vi "iWorx - Conductivity_.vi"() -> ()   [LabVIEW 2012]
uses:
  <vilib>/DAQmx/read.llb/DAQmx Read (Analog 1D Wfm NChan 1Samp).vi
  <vilib>/DAQmx/create/channels.llb/DAQmx Create Channel (AI-Voltage-Basic).vi
  <vilib>/DAQmx/miscellaneous.llb/DAQmx Fill In Error Info.vi
panel:
  in  "Reset Default Cal":bool
  in  "Set Points":T1={"SP1 Voltage"=0.2, "SP1 Value"=20.0, "SP1 Voltage 2"=2.0, "SP1 Value 2"=200.0} {"SP1 Value 2" format="%.1f mS"; "SP1 Voltage 2" format="%.1f V"; "SP1 Value" format="%.1f mS"; "SP1 Voltage" format="%.1f V"}
  in  "Set Up":bool
  out "Offset":dbl=-1.1111111111111112
  out "Slope":dbl=5.277777777777778
  in  "Channel":u16(ring) items=["Channel 1", "Channel 2"]
  in  "Pause Button":bool
  in  "Snapshot":bool
  out "Processed Signal":dbl(knob) caption="Conductivity" scale=0.0..20.0
  in  "stop":bool
  out "Waveform Chart":waveform(dbl)(graph)
  in  "Sample Timing":u16(ring)=200 items=["20Hz"=50, "5 Hz"=200, "2 Hz"=500, "1 Hz"=1000, ".5 Hz"=2000, ".2 Hz"=5000]
  in  "Clear Chart":bool
  in  "Open Log":bool
  in  "Autoscale Y":bool
  out "Raw Signal":dbl(knob) scale=-10.0..10.0
  # "iWorx - Conductivity Probe - Data Logger"
  # "Sensor Input"
  # "(              ,              )"
  # "(              ,              )"
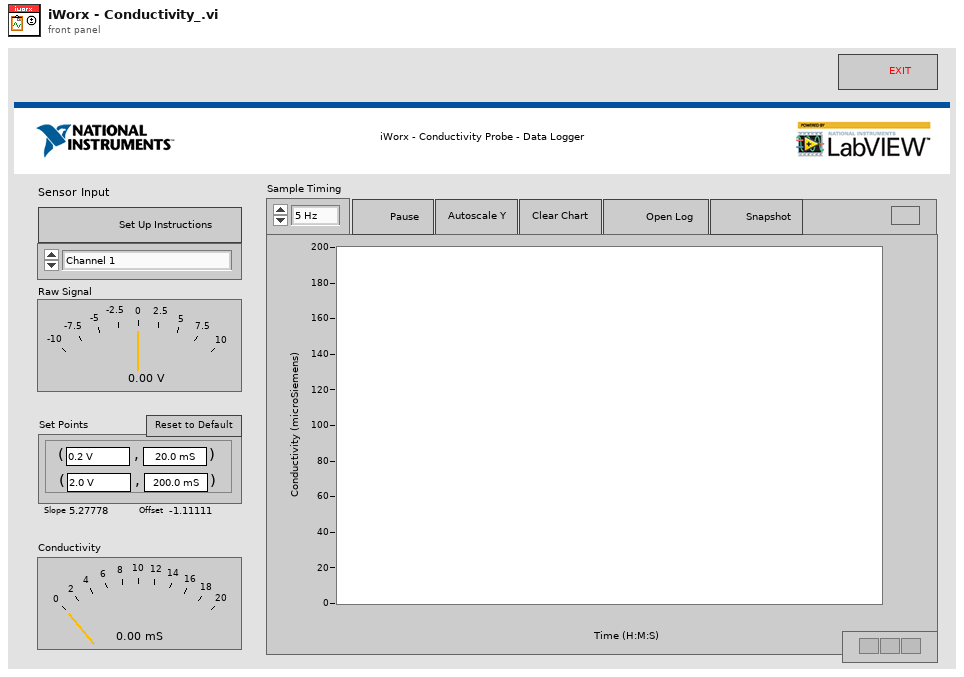
[diagram p1: front panel]
types:
  T1 = cluster{"SP1 Voltage":dbl, "SP1 Value":dbl, "SP1 Voltage 2":dbl, "SP1 Value 2":dbl}
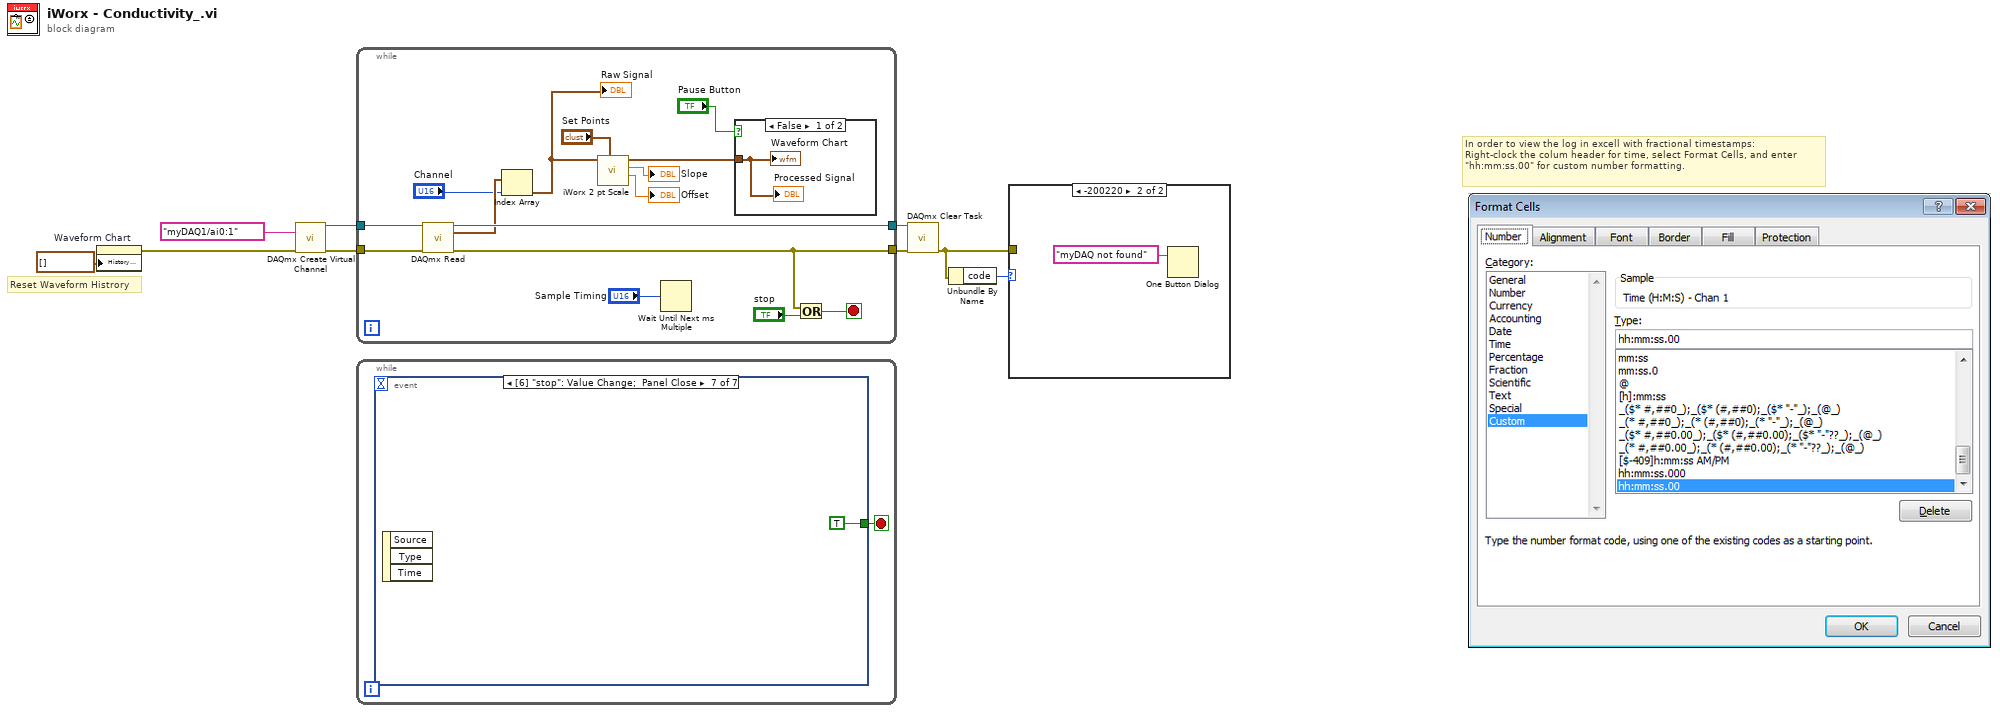
[diagram p0: block diagram]
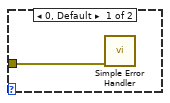
[diagram p2: hidden frame]
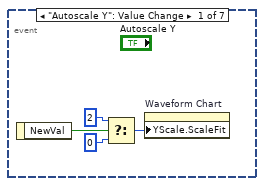
[diagram p3: hidden frame]
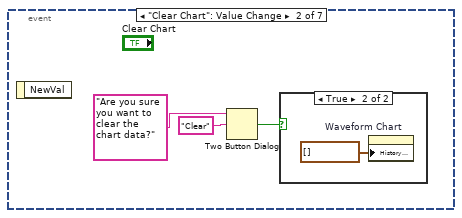
[diagram p4: hidden frame]
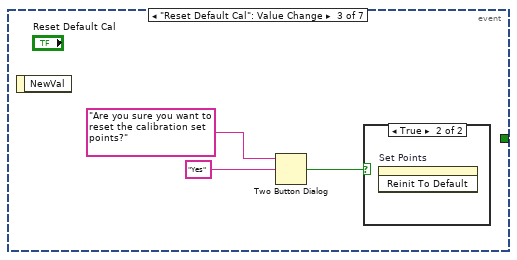
[diagram p6: hidden frame]
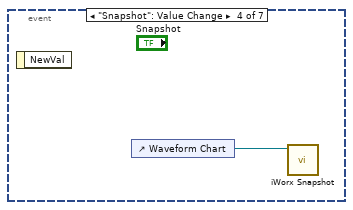
[diagram p8: hidden frame]
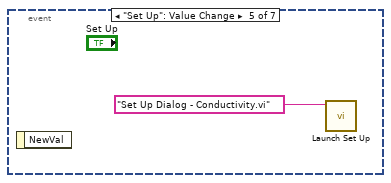
[diagram p9: hidden frame]
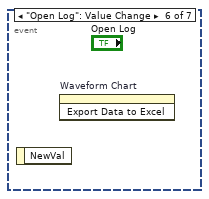
[diagram p10: hidden frame]
diagram:
  # "Reset Waveform Histrory"
  # "In order to view the log in excell with fractional timestamps: \nRight-clock the colum header for time, select Format Cells, and enter \"hh:mm:ss.00\" for custom number formatting."
  n1 = property on="Waveform Chart" class="WFChart (strict)"("History Data"=waveform(dbl)[] []) -> (error out=w3:errorcluster)  [unwired: 2 in, 1 out]
  n2 = call-poly <vilib>:"DAQmx Create Virtual Channel.vi"("physical channels"=tag "myDAQ1/ai0:1", "error in"=w3) -> ("task out"=w6:refnum<k21>, "error out"=w5:errorcluster)  [unwired: 12 in]
  n3 = while {
    tunnel: w6 -> [w22]
    tunnel: [w21] -> w9
    tunnel: w5 -> [w20]
    tunnel: [w18] -> w8
    stop <- w19 stop-if-true
    n4 = call-poly <vilib>:"DAQmx Read.vi"("task/channels in"=w22, "error in"=w20) -> ("task out"=w21:refnum<k21>, "data"=w16:waveform(dbl)[], "error out"=w18:errorcluster)  [unwired: 11 in]
    n5 = Index Array(array=w16, index="Channel") -> (element=w14:waveform(dbl))
    "Raw Signal" <- w14
    n6 = call "iWorx 2 pt Scale.vi"("Calibration Data"="Set Points", "Raw Waveform"=w14) -> ("Offset"=→"Offset":dbl, "Slope"=→"Slope":dbl, "Scaled Value"=w15:waveform(dbl))  [unwired: 7 in]
    n7 = Wait Until Next ms Multiple(millisecond multiple="Sample Timing") -> ()  [unwired: 1 out]
    n8 = case shown="False" "Pause Button" {
      tunnel: w15 -> [w25 _]
      frame False {
        "Waveform Chart" <- w25
        "Processed Signal" <- w25
      }
      frame True {
      }
    }
    n9 = Or(x=w18, y="stop") -> (x .or. y?=w19:bool)
  }
  n10 = while {
    stop <- w26 stop-if-true
    n11 = event shown="[6] \"stop\": Value Change;  Panel Close" {
      selector: _ -> [_ _ _ _ _ _ _]
      dyn-events: _ -> [_ _ _ _ _ _ _]
      timeout: _ -> [_ _ _ _ _ _ _]
      tunnel: [_ _ _ _ _ _ TRUE] -> w26
      event "Autoscale Y": Value Change {
        n12 = event-data() -> ("NewVal"=w28:bool)  [unwired: 1 in]
        n13 = Select(t=u8 2 ("Y Scale.Scale Fit"), s=w28, f=u8 0 ("Y Scale.Scale Fit")) -> (s? t:f=w27:u8)
        n14 = property on="Waveform Chart" class="WFChart (strict)"("YScale.ScaleFit"=w27) -> ()  [unwired: 2 in, 2 out]
      }
      event "Clear Chart": Value Change {
        n15 = event-data() -> ()  [unwired: 1 in, 1 out]
        n16 = Two Button Dialog(message="Are you sure you want to clear the chart data?", 2:"Clear" ("T button name (\"OK\")")) -> (T button?=w32:bool)  [unwired: 1 in]
        n17 = case shown="True" w32 {
          frame False {
          }
          frame True {
            n18 = property on="Waveform Chart" class="WFChart (strict)"("History Data"=waveform(dbl)[] []) -> ()  [unwired: 2 in, 2 out]
          }
        }
      }
      event "Reset Default Cal": Value Change {
        n19 = event-data() -> ()  [unwired: 1 in, 1 out]
        n20 = Two Button Dialog(message="Are you sure you want to reset the calibration set points?", 2:"Yes" ("T button name (\"OK\")")) -> (T button?=w37:bool)  [unwired: 1 in]
        n21 = case shown="True" w37 {
          frame False {
          }
          frame True {
            n22 = invoke on="Set Points" class="Clust (strict)" method="Reinit To Default"() -> ()  [unwired: 3 in, 3 out]
          }
        }
      }
      event "Snapshot": Value Change {
        n23 = event-data() -> ()  [unwired: 1 in, 1 out]
        n24 = control-ref of="Waveform Chart"() -> (w38:refnum<vi>)
        n25 = call "iWorx Snapshot.vi"("WaveformChart in"=w38) -> ()  [unwired: 10 in, 1 out]
      }
      event "Set Up": Value Change {
        n26 = event-data() -> ()  [unwired: 1 in, 1 out]
        n27 = call "Launch Set Up.vi"("name or relative path"="Set Up Dialog - Conductivity.vi") -> ()  [unwired: 9 in, 2 out]
      }
      event "Open Log": Value Change {
        n28 = event-data() -> ()  [unwired: 1 in, 1 out]
        n29 = invoke on="Waveform Chart" class="WFChart (strict)" method="Export Data to Excel"() -> ()  [unwired: 3 in, 3 out]
      }
      event "stop": Value Change; Panel Close {
        n30 = event-data() -> ()  [unwired: 1 in, 3 out]
      }
    }
  }
  n31 = call <vilib>:"DAQmx Clear Task.vi"("task in"=w9, "error in"=w8) -> ("error out"=w1:errorcluster)  [unwired: 13 in]
  n32 = Unbundle By Name(w1) -> ("code"=w2:i32)
  n33 = case shown="-200220" w2 {
    tunnel: w1 -> [w41 _]
    frame 0, Default {
      n34 = call <vilib>:"Simple Error Handler.vi"("error in (no error)"=w41) -> ()  [unwired: 4 in, 5 out]
    }
    frame -200220 {
      n35 = One Button Dialog(message="myDAQ not found") -> ()  [unwired: 1 in, 1 out]
    }
  }
